vi "Amplitude Modulation and Demodulation.vi"() -> ()   [LabVIEW 2013]
uses:
  <vilib>/sound2/lvsound2.llb/Sound File Info (path).vi
  <vilib>/sound2/lvsound2.llb/Sound File Read Open.vi
  <vilib>/sound2/lvsound2.llb/Sound File Read (DBL).vi
  <vilib>/Waveform/WDTOps.llb/WDT Get Waveform Subset DBL.vi
  <vilib>/express/express analysis/Spectral/Block/exnSpectralBlock spectral measurements power poly.vi
  <vilib>/express/express analysis/Spectral/Block/exnSpectralBlock spectral measurements power DDT.vi
  <vilib>/express/express analysis/Spectral/Block/exnSpectralBlock spectral measurements RMS poly.vi
  <vilib>/express/express analysis/Spectral/Block/exnSpectralBlock spectral measurements RMS DDT.vi
  <vilib>/express/express analysis/Spectral/XNode/ExpressSpectralMeasurementsBlockNode.xnode
panel:
  in  "Wait Interval (ms)":dbl=1500.0
  in  "Modulated Signal Source":enum32{"Single Tone", "From File"}(tab)
  in  "ST Frequency":dbl=2000.0 caption="Frequency"
  in  "ST Amplitude":dbl=1.0 caption="Amplitude"
  in  "Resample Rate":dbl=1000000.0 format="%#_6f"
  in  "Duration":dbl=44100.0
  in  "WAV Path":path caption="Path"
  out "After Rectifier":dynamicdata(graph)
  out "AM Power Specturm":dynamicdata(graph)
  out "After Filter":dynamicdata(graph)
  in  "WAV Sample Rate":dbl=44100.0 caption="Output Sample Rate"
  in  "LPF Cut-Off":dbl=10000.0 caption="Cut-off Frequency"
  in  "SNR (dB)":dbl(slide)=0.6 caption="Standard deviation" scale=-20.0..30.0
  out "Comparision":dynamicdata(graph) caption="Demodulated Wave"
  out "Baseband":dynamicdata(graph)
  out "AM FFT":dynamicdata(graph)
  out "AM Wave":dynamicdata(graph)
  in  "DC Offset":dbl=1.0 caption="Carrier DC Offset"
  in  "Carrier Amp.":dbl=1.0 caption="Carrier Amplitude"
  in  "Stop":bool
  in  "Modulation Index":dbl(slide)=1.0 scale=0.0..5.0
  in  "Carrier Freq.":dbl=10000.0 caption="Carrier Frequency" format="%#_6f"
  # "Amplitude Modulation"
  # "Baseband"
  # "Modulation"
  # "Demodulation"
  # "注：由于配置原因，噪声采样率为 1000000 时，样本数超过 100000 即会崩溃，导致音频最多保留 0.1s。为了延长音频时间，便于查看效果，此处将默认的采样频率由 1000000 降低至 100000，载波频率降低至 20000。"
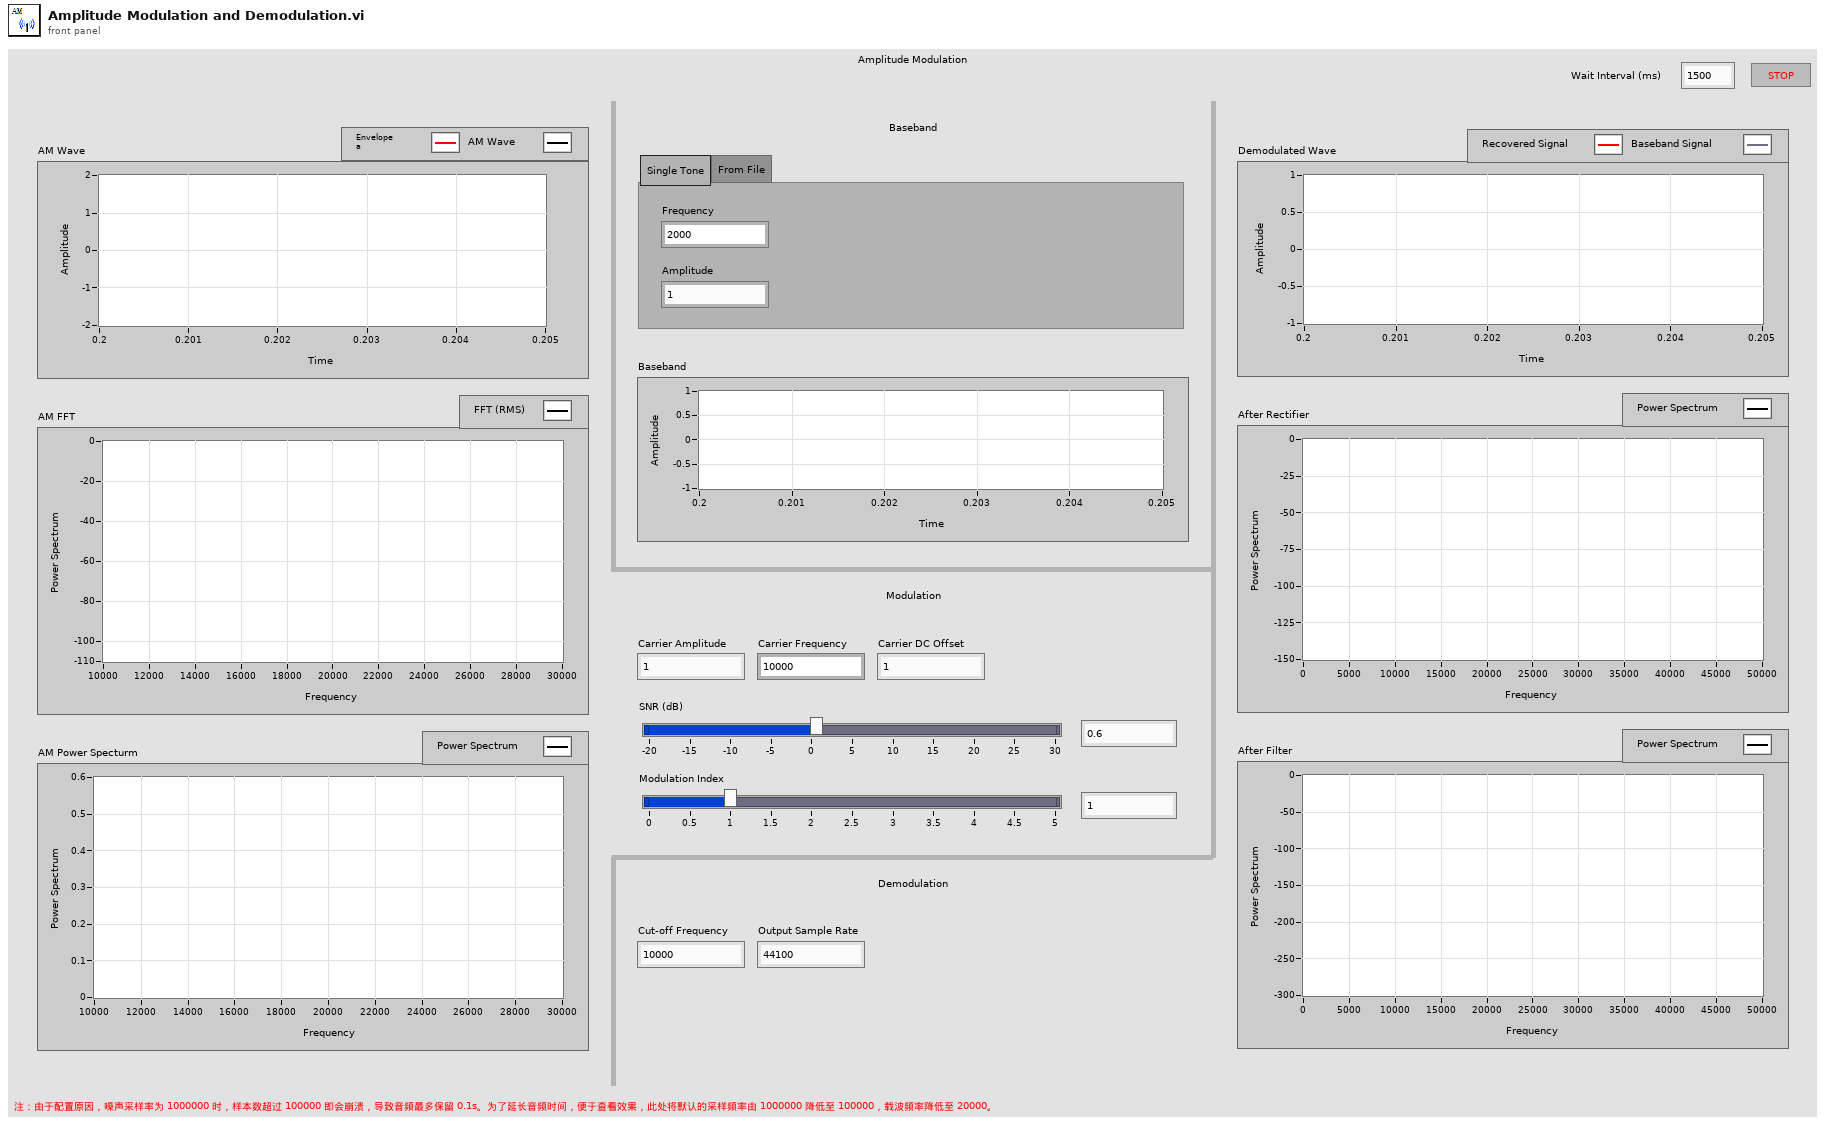
[diagram p1: front panel]
types:
  T1 = typedef "Sound File Refnum.ctl" = refnum<file>
  T2 = cluster{"averaging mode":u16, "weighting mode":u16, "number of averages":u32}
  T3 = cluster{"dB On (F)":bool, "unwrap phase (F)":bool, "convert to degree (F)":bool}
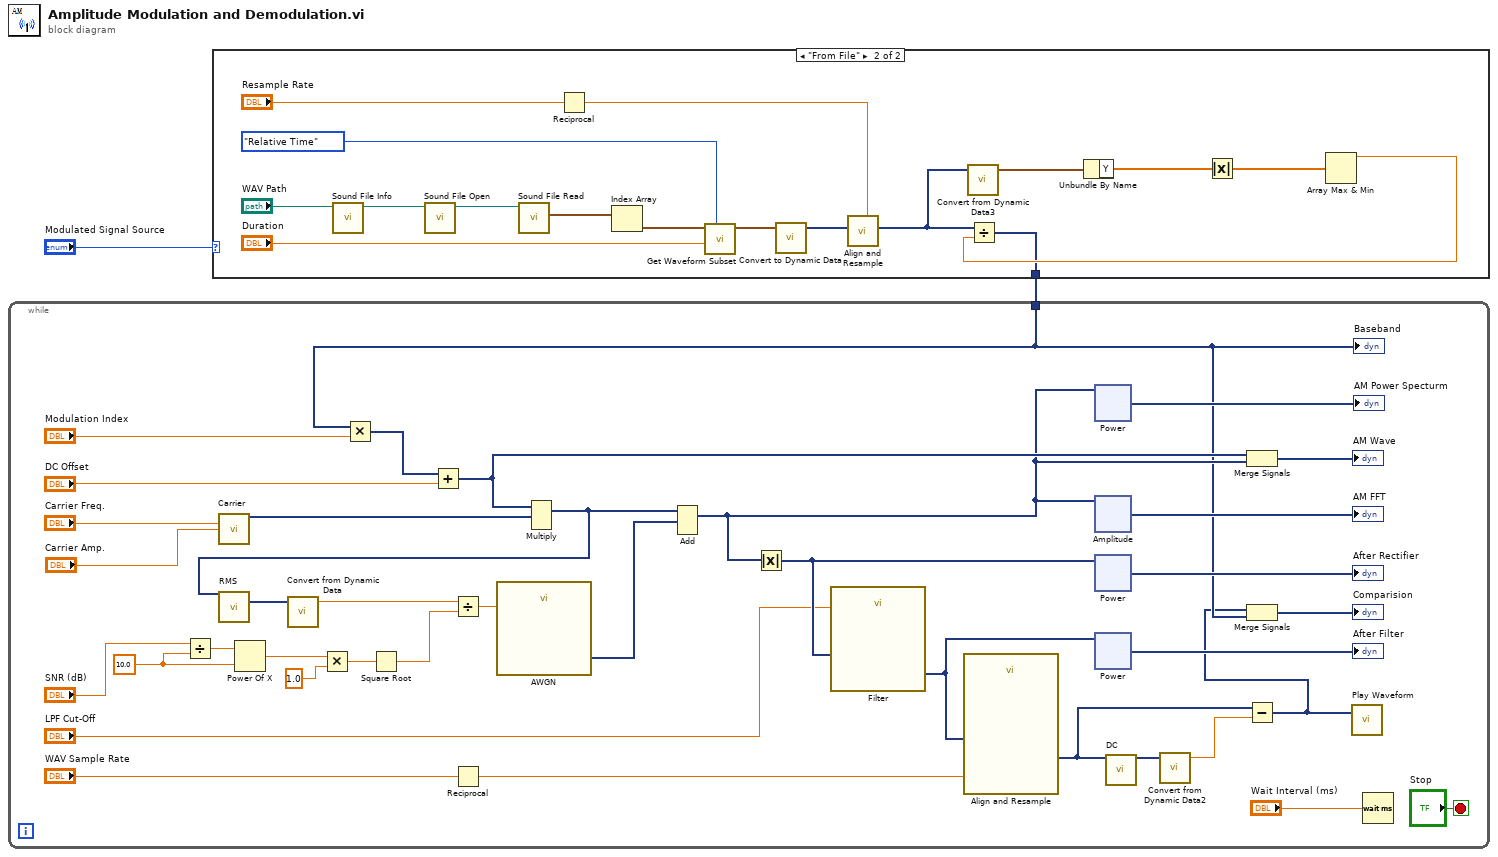
[diagram p0: block diagram]
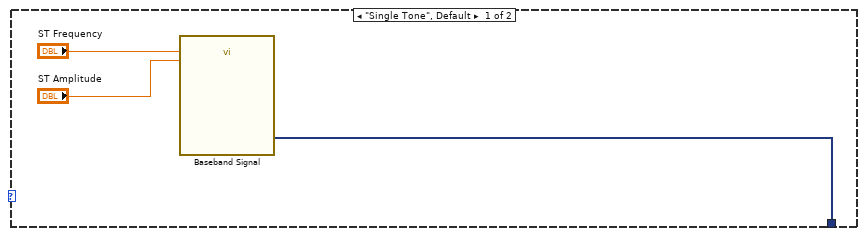
[diagram p2: hidden frame]
diagram:
  n1 = case shown="\"From File\"" "Modulated Signal Source" {
    tunnel: [w3 w7] -> w1
    frame "Single Tone", Default {
      n2 = call "Baseband Signal"("Frequency"="ST Frequency", "Amplitude"="ST Amplitude") -> ("Sine"=w3:dynamicdata)  [unwired: 12 in, 1 out]
    }
    frame "From File" {
      n3 = call-poly <vilib>:"Sound File Info.vi"("path"="WAV Path") -> ("path out"=w20:path)  [unwired: 7 in, 3 out]
      n4 = call-poly <vilib>:"Sound File Open.vi"("path"=w20) -> ("sound file refnum"=w22:T1)  [unwired: 9 in, 1 out]
      n5 = call-poly <vilib>:"Sound File Read.vi"("sound file refnum"=w22) -> ("data"=w17:waveform(dbl)[])  [unwired: 6 in, 4 out]
      n6 = Reciprocal(x="Resample Rate") -> (1/x=w13:dbl)
      n7 = Index Array(array=w17) -> (element=w18:waveform(dbl))  [unwired: 1 in]
      n8 = call-poly <vilib>:"Get Waveform Subset.vi"("start/duration format"=enum16{"Relative Time"}."Relative Time", "duration"="Duration", "waveform in"=w18) -> ("waveform out"=w12:waveform(dbl))  [unwired: 3 in, 3 out]
      n9 = call "Convert to Dynamic Data"("Waveform"=w12) -> ("Dynamic Data Type"=w6:dynamicdata)  [unwired: 3 in]
      n10 = call "Align and Resample"("dt"=w13, "Signals"=w6) -> ("Resampled Signals"=w8:dynamicdata)  [unwired: 7 in, 2 out]
      n11 = call "Convert from Dynamic Data3"("Dynamic Data Type"=w8) -> ("Waveform"=w15:waveform(dbl))  [unwired: 3 in]
      n12 = Unbundle By Name(w15) -> ("Y"=w9:dbl[])
      n13 = Absolute Value(x=w9) -> (abs(x)=w11:dbl[])
      n14 = Array Max & Min(array=w11) -> (max value=w10:dbl)  [unwired: 3 out]
      n15 = Divide(x=w8, y=w10) -> (x/y=w7:dynamicdata)
    }
  }
  n16 = while {
    tunnel: w1 -> [w27]
    stop <- "Stop" stop-if-true
    w48 = 10.0
    n17 = Divide(x="SNR (dB)", y=w48) -> (x/y=w47:dbl)
    n18 = call "Carrier"("Frequency"="Carrier Freq.", "Amplitude"="Carrier Amp.") -> ("Sine"=w54:dynamicdata)  [unwired: 12 in, 1 out]
    n19 = Power Of X(1:w48, 2:w47) -> (0:w46:dbl)
    n20 = Multiply(x=w46, y=1.0) -> (x*y=w44:dbl)
    n21 = Multiply(x=w27, y="Modulation Index") -> (x*y=w52:dynamicdata)
    n22 = Square Root(x=w44) -> (sqrt(x)=w43:dbl)
    n23 = Add(x=w52, y="DC Offset") -> (x+y=w51:dynamicdata)
    n24 = Reciprocal(x="WAV Sample Rate") -> (1/x=w32:dbl)
    n25 = Multiply(1:w54, 2:w51) -> (0:w40:dynamicdata)  [unwired: 1 in, 1 out]
    n26 = call "RMS"("Signals"=w40) -> ("RMS"=w49:dynamicdata)  [unwired: 13 in, 1 out]
    n27 = call "Convert from Dynamic Data"("Dynamic Data Type"=w49) -> ("Scalar"=w42:dbl)  [unwired: 3 in]
    n28 = Divide(x=w42, y=w43) -> (x/y=w41:dbl)
    n29 = call "AWGN"("Standard deviation"=w41) -> ("DC with Gaussian Noise"=w23:dynamicdata)  [unwired: 13 in, 1 out]
    n30 = Add(1:w23, 2:w40) -> (0:w29:dynamicdata)  [unwired: 1 in, 1 out]
    n31 = Absolute Value(x=w29) -> (abs(x)=w36:dynamicdata)
    n32 = call "Filter"("Lower Cut-Off"="LPF Cut-Off", "Signal"=w36) -> ("Filtered Signal"=w24:dynamicdata)  [unwired: 8 in, 1 out]
    n33 = call "Align and Resample"("dt"=w32, "Signals"=w24) -> ("Resampled Signals"=w34:dynamicdata)  [unwired: 7 in, 2 out]
    n34 = xnode "Power"("Signals"=w29) -> ("Power Spectrum"=→"AM Power Specturm":dynamicdata)  [unwired: 1 in, 1 out]
    n35 = xnode "Amplitude"("Signals"=w29) -> ("FFT - (RMS)"=→"AM FFT":dynamicdata)  [unwired: 1 in, 2 out]
    n36 = xnode "Power"("Signals"=w36) -> ("Power Spectrum"=→"After Rectifier":dynamicdata)  [unwired: 1 in, 1 out]
    n37 = xnode "Power"("Signals"=w24) -> ("Power Spectrum"=→"After Filter":dynamicdata)  [unwired: 1 in, 1 out]
    n38 = call "DC"("Signals"=w34) -> ("Mean (DC)"=w38:dynamicdata)  [unwired: 13 in, 1 out]
    n39 = call "Convert from Dynamic Data2"("Dynamic Data Type"=w38) -> ("Scalar"=w37:dbl)  [unwired: 3 in]
    n40 = Merge Signals(w51, w29) -> (→"AM Wave":dynamicdata)
    n41 = Subtract(x=w34, y=w37) -> (x-y=w25:dynamicdata)
    n42 = Merge Signals(w25, w27) -> (→"Comparision":dynamicdata)
    n43 = call "Play Waveform"("Data"=w25) -> ()  [unwired: 18 in, 1 out]
    n44 = Wait (ms)(milliseconds to wait="Wait Interval (ms)") -> ()  [unwired: 1 out]
    "Baseband" <- w27
  }
